vi "Ny_ekg.vi"() -> ()   [LabVIEW 2016]
uses:
  <vilib>/Utility/file.llb/Write Delimited Spreadsheet (DBL).vi
panel:
  out "Pulse Led":bool
  in  "stop measurement":bool
  out "Periode":dbl format="%#_3f"
  out "Pulse":dbl format="%#_3f"
  in  "Tab Control 2":enum32{"Main", "Simulering", "Filter", "Peak"}(tab)
  in  "Fil Navn":string="Auto_dump"
  out "Pulse graph":dbl(graph)
  in  "Save data":bool
  in  "Enum":enum16{"Real signal", "Simulation"}(ring)
  in  "block size":dbl=1.0
  in  "sampling rate":dbl=1000.0
  in  "Save  sim og ekte":bool
  in  "Hardware":bool
  out "EKG in og ut":dynamicdata(graph)
  in  "Lavpass":bool
  in  "Lower Cut-Off":dbl=35.0
  out "Filtered":dynamicdata(graph)
  in  "High cut-off":dbl(slide)=10.0 caption="Lower Cut-Off" scale=0.1..1.0
  in  "Filter":bool
  in  "Høypass":bool
  in  "Bot value":dbl(slide) scale=-1.0..1.0
  in  "Top value":dbl(slide)=1.5 scale=0.0..2.0
  in  "Sample Rate":dbl=1000.0 format="%#_13g"
  out "Raw Input data":dynamicdata(graph)
  out "EKG 2":dynamicdata(graph)
  # "Simulation Settings"
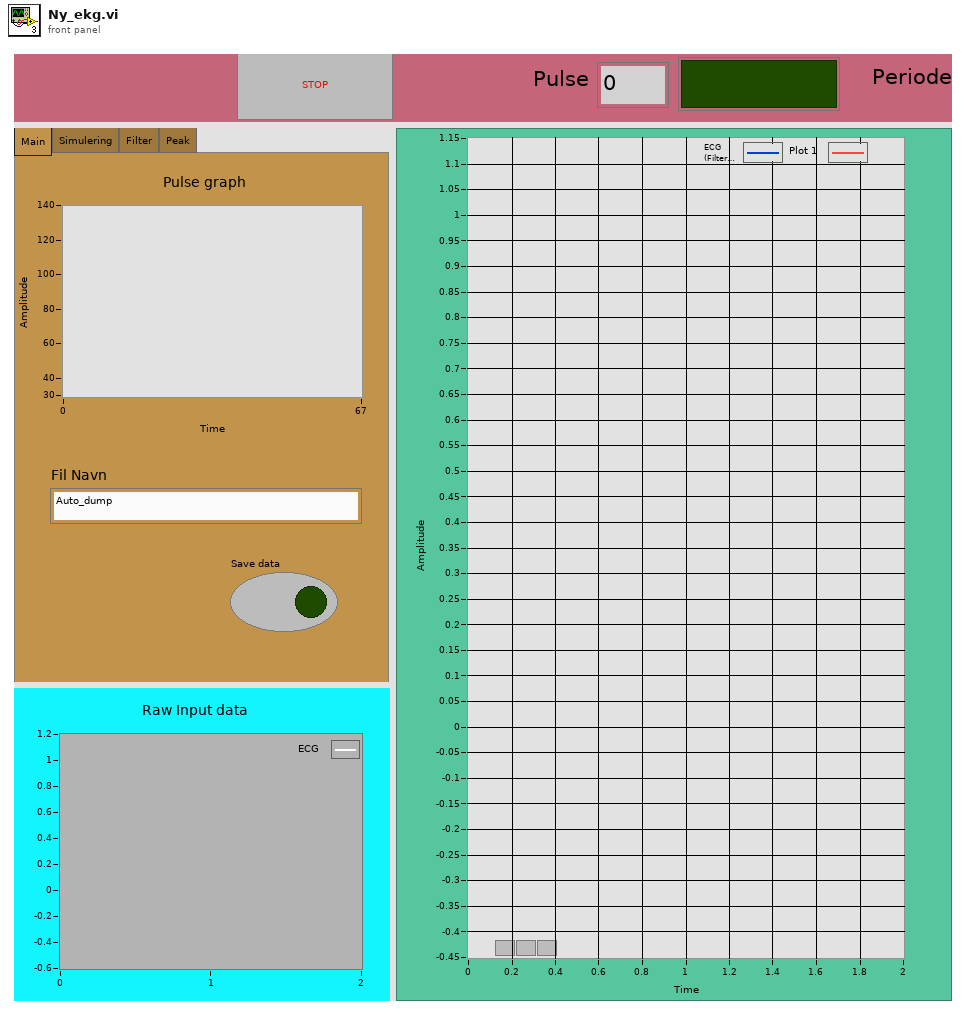
[diagram p1: front panel]
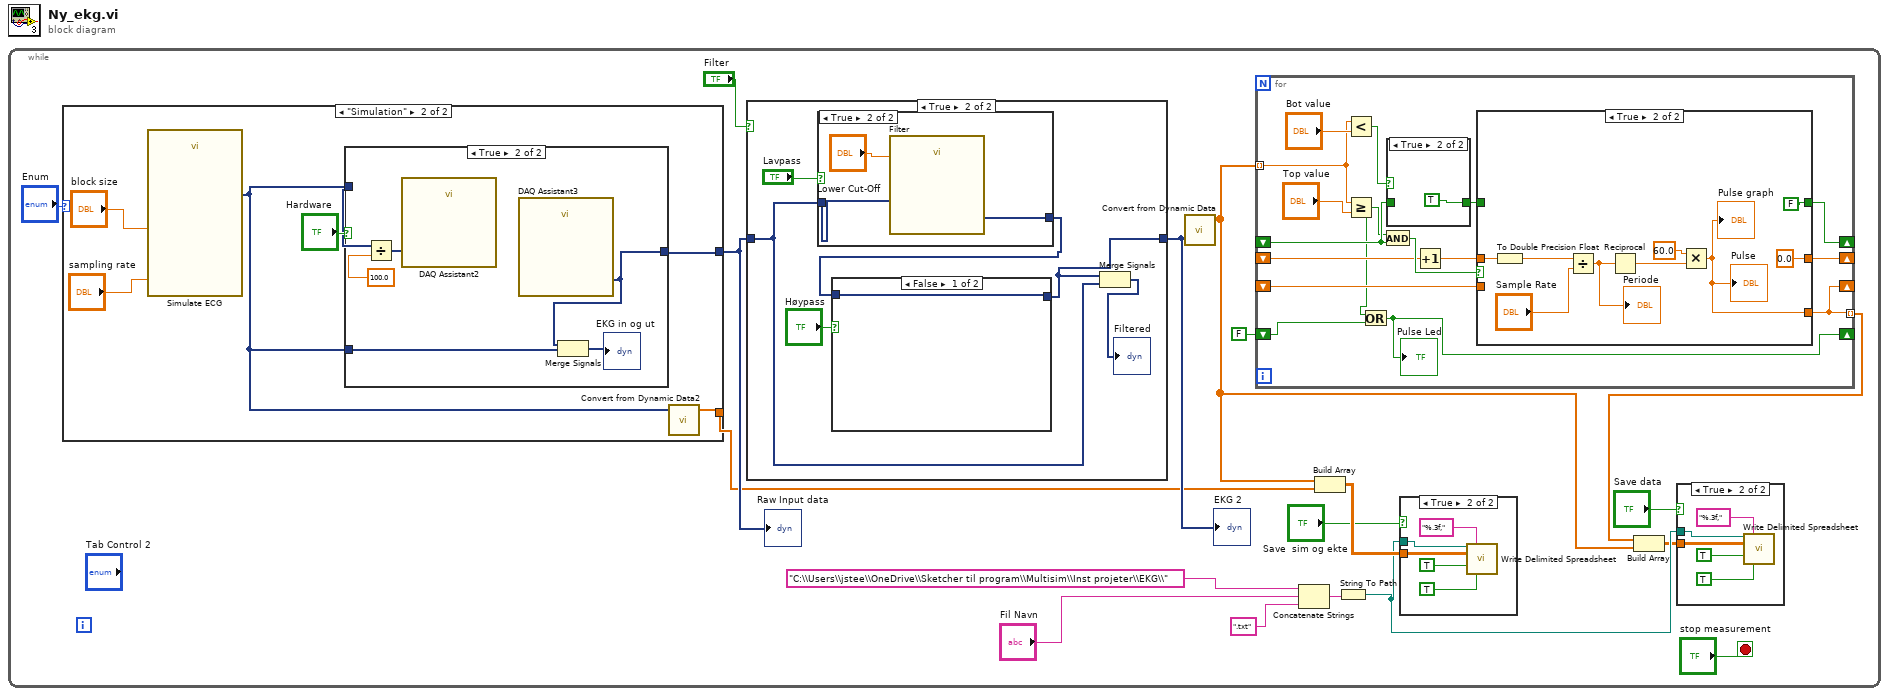
[diagram p0: block diagram]
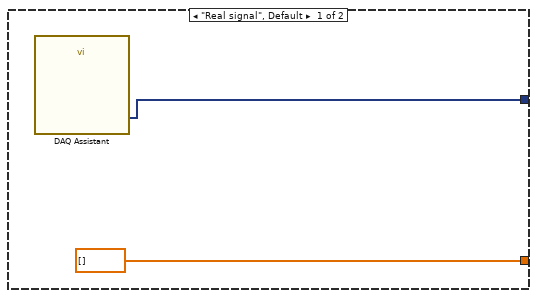
[diagram p4: hidden frame]
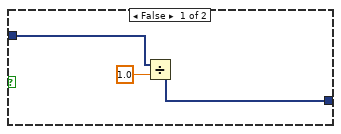
[diagram p5: hidden frame]
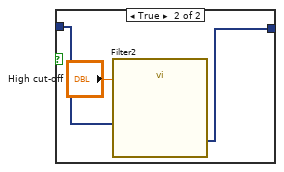
[diagram p7: hidden frame]
diagram:
  n1 = while {
    stop <- "stop measurement" stop-if-true
    n2 = case shown="\"Simulation\"" "Enum" {
      tunnel: [w30 w33] -> w16
      tunnel: [dbl[] [] ("Array") w32] -> w8
      frame "Real signal", Default {
        n3 = call "DAQ Assistant"() -> ("data"=w30:dynamicdata)  [unwired: 16 in, 3 out]
      }
      frame "Simulation" {
        n4 = call "Simulate ECG"("sampling rate"="sampling rate", "block size"="block size") -> ("ECG"=w31:dynamicdata)  [unwired: 8 in, 1 out]
        n5 = case shown="True" "Hardware" {
          tunnel: w31 -> [w38 w45]
          tunnel: [w39 w40] -> w33
          tunnel: w31 -> [_ w42]
          frame False {
            n6 = Divide(x=w38, y=1.0) -> (x/y=w39:dynamicdata)
          }
          frame True {
            n7 = Divide(x=w45, y=100.0) -> (x/y=w43:dynamicdata)
            n8 = call "DAQ Assistant2"("data"=w43) -> ()  [unwired: 16 in, 3 out]
            n9 = call "DAQ Assistant3"() -> ("data"=w40:dynamicdata)  [unwired: 16 in, 3 out]
            n10 = Merge Signals(w40, w42) -> (→"EKG in og ut":dynamicdata)
          }
        }
        n11 = call "Convert from Dynamic Data2"("Dynamic Data Type"=w31) -> ("Array"=w32:dbl[])  [unwired: 3 in]
      }
    }
    "Raw Input data" <- w16
    n12 = case shown="True" "Filter" {
      tunnel: w16 -> [w46 w51]
      tunnel: [w46 w47] -> w15
      frame False {
      }
      frame True {
        n13 = case shown="True" "Lavpass" {
          tunnel: [w57 w59] -> w48
          tunnel: w51 -> [w57 w58]
          frame False {
          }
          frame True {
            n14 = call "Filter"("Lower Cut-Off"="Lower Cut-Off", "Signal"=w58) -> ("Filtered Signal"=w59:dynamicdata)  [unwired: 8 in, 1 out]
          }
        }
        n15 = case shown="False" "Høypass" {
          tunnel: w48 -> [w53 w56]
          tunnel: [w53 w55] -> w47
          frame False {
          }
          frame True {
            n16 = call "Filter2"("Lower Cut-Off"="High cut-off", "Signal"=w56) -> ("Filtered Signal"=w55:dynamicdata)  [unwired: 8 in, 1 out]
          }
        }
        n17 = Merge Signals(w47, w51) -> (→"Filtered":dynamicdata)
      }
    }
    "EKG 2" <- w15
    n18 = call "Convert from Dynamic Data"("Dynamic Data Type"=w15) -> ("Array"=w6:dbl[])  [unwired: 3 in]
    n19 = for {
      tunnel: w6 -> [w75] mode=indexing
      shift-right: [w72] -> _
      shift-left: _ -> [w64]
      shift-right: [w67] -> _
      shift-left: _ -> [w69]
      tunnel: [w66] -> w7 mode=indexing
      shift-right: [w66] -> _
      shift-left: _ -> [w65]
      shift-right: [w61] -> _
      shift-left: FALSE -> [w62]
      n20 = Less?(x=w75, y="Bot value") -> (x < y?=w74:bool)
      n21 = Greater Or Equal?(x=w75, y="Top value") -> (x >= y?=w63:bool)
      n22 = Or(x=w63, y=w62) -> (x .or. y?=w61:bool)
      "Pulse Led" <- w61
      n23 = And(x=w63, y=w64) -> (x .and. y?=w71:bool)
      n24 = case shown="True" w74 {
        tunnel: [w77 TRUE] -> w73
        tunnel: w64 -> [w77 _]
        frame False {
        }
        frame True {
        }
      }
      n25 = Increment(x=w69) -> (x+1=w68:dbl)
      n26 = case shown="True" w71 {
        tunnel: w73 -> [w81 _]
        tunnel: [w81 FALSE] -> w72
        tunnel: w68 -> [w80 w85]
        tunnel: [w80 0.0] -> w67
        tunnel: [w79 w82] -> w66
        tunnel: w65 -> [w79 _]
        frame False {
        }
        frame True {
          n27 = To Double Precision Float(number=w85) -> (double precision float=w86:dbl)
          n28 = Divide(x=w86, y="Sample Rate") -> (x/y=w87:dbl)
          "Periode" <- w87
          n29 = Reciprocal(x=w87) -> (1/x=w83:dbl)
          n30 = Multiply(x=60.0 ("x*y"), y=w83) -> (x*y=w82:dbl)
          "Pulse" <- w82
          "Pulse graph" <- w82
        }
      }
    }
    n31 = Concatenate Strings("C:\\Users\\jstee\\OneDrive\\Sketcher til program\\Multisim\\Inst projeter\\EKG\\", "Fil Navn", ".txt" ("string")) -> (w14:string)
    n32 = Build Array(w6, w8) -> (w10:dbl[][])
    n33 = String To Path(string=w14) -> (path=w4:path)
    n34 = case shown="True" "Save  sim og ekte" {
      tunnel: w10 -> [_ w25]
      tunnel: w4 -> [_ w24]
      frame False {
      }
      frame True {
        n35 = call-poly <vilib>:"Write Delimited Spreadsheet.vi"("file path (dialog if empty)"=w24, "format (%.3f)"="%.3f,", "2D data"=w25, "append to file? (new file:F)"=TRUE, "transpose? (no:F)"=TRUE) -> ()  [unwired: 9 in, 2 out]
      }
    }
    n36 = Build Array(w7, w6) -> (w3:dbl[][])
    n37 = case shown="True" "Save data" {
      tunnel: w4 -> [_ w20]
      tunnel: w3 -> [_ w19]
      frame False {
      }
      frame True {
        n38 = call-poly <vilib>:"Write Delimited Spreadsheet.vi"("file path (dialog if empty)"=w20, "format (%.3f)"="%.3f,", "2D data"=w19, "append to file? (new file:F)"=TRUE, "transpose? (no:F)"=TRUE) -> ()  [unwired: 9 in, 2 out]
      }
    }
  }
